vi "Ctor.vi"(8 "error in (no error)":errorcluster, 9 "Is Scrollback? (F)":bool, 10 "Rows (24)":i32=24, 11 "Cols (80)":i32=80) -> (0 "error out":errorcluster, 3 "TermBuffer out":refnum<class "TermBuffer.lvclass">)   [LabVIEW 2020, in "Terminal.lvlib" / "TermBuffer.lvclass"]
uses:
  TermBuffer.lvclass
  TermBuffer.lvclass/TermBuffer.ctl
  TermLine/TermLine.lvclass
  Ref Data.ctl
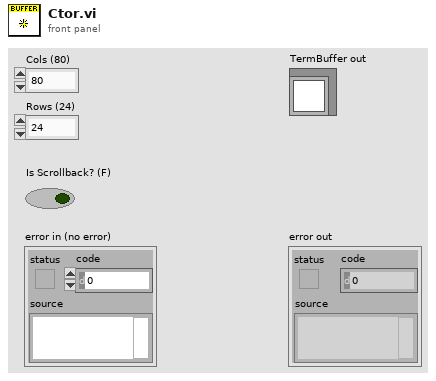
[diagram p1: front panel]
types:
  T1 = typedef "Terminal.lvlib/TermBuffer.lvclass/Ref Data.ctl" = cluster{"Lines":refnum<class "TermLine.lvclass">[], "Rows":i32, "Cols":i32}
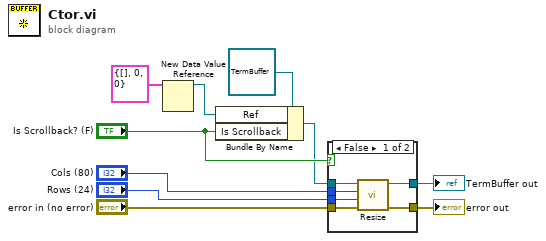
[diagram p0: block diagram]
diagram:
  n1 = New Data Value Reference(data value=T1 {"Lines"=[], "Rows"=0, "Cols"=0} ("Ref Data")) -> (data value reference=w2:refnum<data-value>)  [unwired: 1 in, 1 out]
  n2 = Bundle By Name(cluster=refnum<class "TermBuffer.lvclass"> refnum ("TermBuffer in"), "Ref"=w2, "Is Scrollback"="Is Scrollback? (F)") -> (w1:refnum<class "TermBuffer.lvclass">)
  n3 = case shown="False" "Is Scrollback? (F)" {
    tunnel: [w16 w18] -> w8
    tunnel: [w15 w17] -> w7
    tunnel: w1 -> [w14 w18]
    tunnel: "error in (no error)" -> [w13 w17]
    tunnel: "Rows (24)" -> [w11 _]
    tunnel: "Cols (80)" -> [w12 _]
    frame False {
      n4 = call "Resize.vi"("error in (no error)"=w13, "Rows"=w11, "Cols"=w12, "TermBuffer in"=w14) -> ("error out"=w15:errorcluster, "TermBuffer out"=w16:refnum<class "TermBuffer.lvclass">)  [unwired: 6 in]
    }
    frame True {
    }
  }
  "error out" <- w7
  "TermBuffer out" <- w8
